vi "Write write delay (ms).vi"(10 "write delay (ms)":i32=-1, 11 "ConfigManager.Text in":refnum<class "ConfigManager.Text.lvclass">) -> (3 "ConfigManager.Text out":refnum<class "ConfigManager.Text.lvclass">)   [LabVIEW 2013, in "CfgManager.Text.lvlib" / "ConfigManager.Text.lvclass"]
doc: "Write Delay (ms) instructs the process to delay the saving to file of a change by a certain number of milliseconds. This allows multiple consecutive changes to be concatenetad into a single Write operation.\n\n-1: Never write to file (unless specifically requested by a Save command)\n0: Write to file immediately\n>1: Apply delay"
uses:
  ConfigManager.Text.lvclass
  ConfigManager.Text.lvclass/ConfigManager.Text.ctl
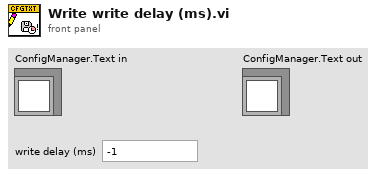
[diagram p1: front panel]
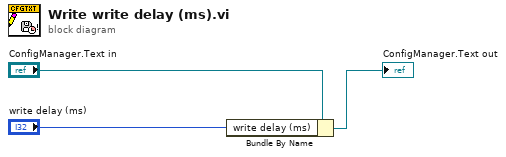
[diagram p0: block diagram]
diagram:
  n1 = Bundle By Name(cluster="ConfigManager.Text in", "write delay (ms)"="write delay (ms)") -> (→"ConfigManager.Text out":refnum<class "ConfigManager.Text.lvclass">)
